vi "oa_Calculate Orbit Precession Direction.vi"(4 "revolutions":dbl format="%.2f", 5 "reset? (F)":bool, 6 "actual samples/rev":dbl format="%.2f", 7 "tach duty":i32=1, 8 "error in (no error)":errorcluster, 9 "max axis value":dbl format="%.2f", 10 "shaft rotating direction":u16, 11 "XY plot data in":cluster{dbl[], dbl[]}[](array[cluster]) {"?" format="%.2f"; "?" format="%.2f"}) -> (0 "error out":errorcluster, 1 "max value":dbl, 2 "orbit precession direction":u16(ring) items=["forward", "backward"], 3 "XY plot data out":cluster{dbl[], dbl[]}[](array[cluster]) {"?" format="%.2f"; "?" format="%.2f"})   [LabVIEW 2017]
uses:
  <vilib>/Analysis/1siggen.llb/Ramp Pattern by Samples.vi
  <vilib>/Analysis/NI_AALPro.lvlib
  <vilib>/Analysis/NI_AALBase.lvlib
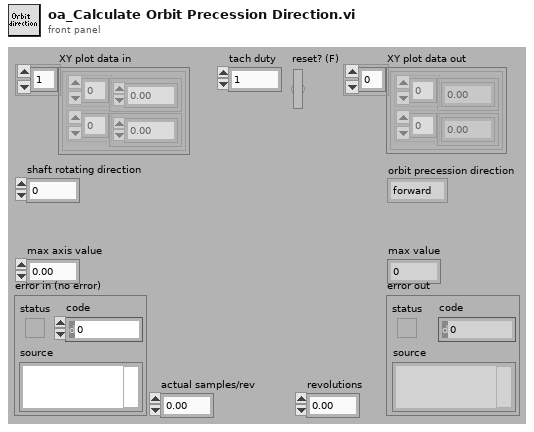
[diagram p1: front panel]
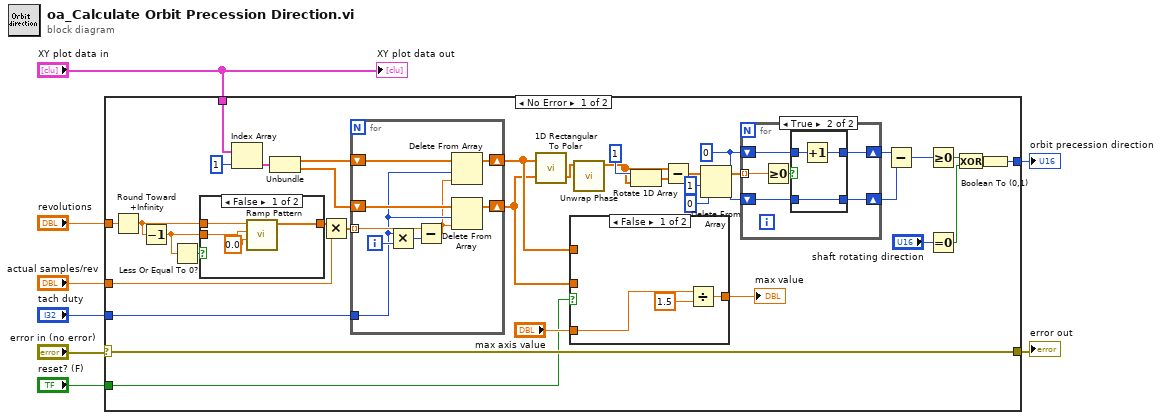
[diagram p0: block diagram]
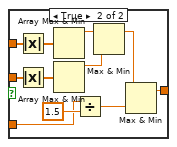
[diagram p2: hidden frame]
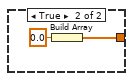
[diagram p3: hidden frame]
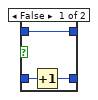
[diagram p4: hidden frame]
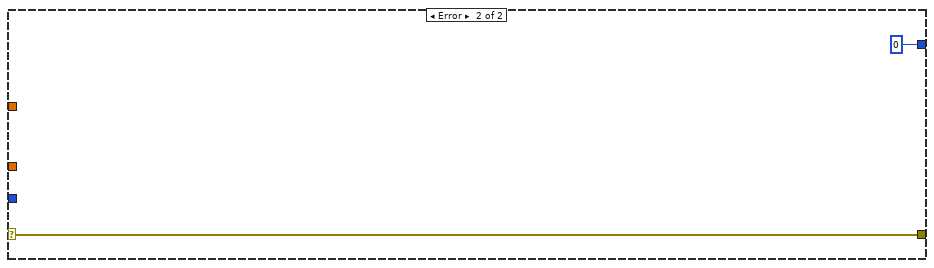
[diagram p5: hidden frame]
diagram:
  n1 = case shown="No Error" "error in (no error)" {
    selector: "error in (no error)" -> [w10 w87]
    tunnel: [w44 i16 0] -> w8
    tunnel: "XY plot data in" -> [w39 _]
    tunnel: "revolutions" -> [w24 _]
    tunnel: "tach duty" -> [w23 _]
    tunnel: "actual samples/rev" -> [w21 _]
    tunnel: [w10 w87] -> w2
    tunnel: "reset? (F)" -> [w9 _]
    frame No Error {
      w26 = 0
      n2 = Round Toward +Infinity(x=w24) -> (ceil(x): smallest int >= x=w13:dbl)
      n3 = Decrement(x=w13) -> (x-1=w11:dbl)
      n4 = Less Or Equal To 0?(x=w11) -> (x <= 0?=w12:bool)
      n5 = case shown="False" w12 {
        tunnel: w13 -> [w61 _]
        tunnel: w11 -> [w60 _]
        tunnel: [w59 w64] -> w20
        frame False {
          n6 = call-poly <vilib>:"Ramp Pattern.vi"("start"=0.0, "end"=w60, "samples"=w61) -> ("Ramp Pattern"=w59:dbl[])  [unwired: 7 in, 1 out]
        }
        frame True {
          n7 = Build Array(0.0 ("element")) -> (w64:dbl[])
        }
      }
      n8 = Index Array(array=w39, index=1) -> (element=w35:cluster{dbl[], dbl[]})
      n9 = Unbundle(w35) -> (w22:dbl[], w18:dbl[])
      n10 = Multiply(x=w20, y=w21) -> (x*y=w19:dbl[])
      n11 = for {
        tunnel: w23 -> [w66]
        shift-right: [w72] -> w17
        shift-left: w22 -> [w73]
        tunnel: w19 -> [w71] mode=indexing
        shift-right: [w67] -> w16
        shift-left: w18 -> [w68]
        i -> [w70]
        n12 = Multiply(x=w66, y=w70) -> (x*y=w69:i32)
        n13 = Subtract(x=w71, y=w69) -> (x-y=w65:dbl)
        n14 = Delete From Array(array=w73, length=w66, index=w65) -> (array with subset deleted=w72:dbl[])  [unwired: 1 out]
        n15 = Delete From Array(array=w68, length=w66, index=w65) -> (array with subset deleted=w67:dbl[])  [unwired: 1 out]
      }
      n16 = call <vilib>:"1D Rectangular To Polar.vi"("X"=w17, "Y"=w16) -> ("Phase"=w27:dbl[])  [unwired: 2 out]
      n17 = case shown="False" w9 {
        tunnel: "max axis value" -> [w47 w53]
        tunnel: [w45 w50] -> w36
        tunnel: w17 -> [_ w49]
        tunnel: w16 -> [_ w48]
        frame False {
          n18 = Divide(x=w47, y=1.5) -> (x/y=w45:dbl)
        }
        frame True {
          n19 = Absolute Value(x=w49) -> (abs(x)=w58:dbl[])
          n20 = Absolute Value(x=w48) -> (abs(x)=w57:dbl[])
          n21 = Array Max & Min(array=w58) -> (max value=w56:dbl)  [unwired: 3 out]
          n22 = Array Max & Min(array=w57) -> (max value=w55:dbl)  [unwired: 3 out]
          n23 = Divide(x=w53, y=1.5) -> (x/y=w52:dbl)
          n24 = Max & Min(x=w56, y=w55) -> (max(x,y)=w51:dbl)  [unwired: 1 out]
          n25 = Max & Min(x=w51, y=w52) -> (max(x,y)=w50:dbl)  [unwired: 1 out]
        }
      }
      "max value" <- w36
      n26 = call <vilib>:"Unwrap Phase.vi"("Phase"=w27) -> ("Unwrapped Phase"=w29:dbl[])  [unwired: 9 in, 1 out]
      n27 = Rotate 1D Array(1:w29, 2:1 ("n")) -> (0:w31:dbl[])
      n28 = Subtract(x=w29, y=w31) -> (x-y=w32:dbl[])
      n29 = Delete From Array(array=w32, length=1, index=0) -> (array with subset deleted=w28:dbl[])  [unwired: 1 out]
      n30 = for {
        tunnel: w28 -> [w79] mode=indexing
        shift-right: [w75] -> w15
        shift-left: w26 -> [w77]
        shift-right: [w74] -> w14
        shift-left: w26 -> [w76]
        n31 = Greater Or Equal To 0?(x=w79) -> (x >= 0?=w78:bool)
        n32 = case shown="True" w78 {
          tunnel: w77 -> [w82 w85]
          tunnel: w76 -> [w81 w83]
          tunnel: [w82 w84] -> w75
          tunnel: [w80 w83] -> w74
          frame False {
            n33 = Increment(x=w81) -> (x+1=w80:i32)
          }
          frame True {
            n34 = Increment(x=w85) -> (x+1=w84:i32)
          }
        }
      }
      n35 = Subtract(x=w15, y=w14) -> (x-y=w38:i32)
      n36 = Greater Or Equal To 0?(x=w38) -> (x >= 0?=w41:bool)
      n37 = Equal To 0?(x="shaft rotating direction") -> (x = 0?=w42:bool)
      n38 = Exclusive Or(1:w42, 2:w41) -> (0:w43:bool)
      n39 = Boolean To (0,1)(Boolean=w43) -> (0, 1=w44:i16)
    }
    frame Error {
    }
  }
  "orbit precession direction" <- w8
  "error out" <- w2
  "XY plot data out" <- "XY plot data in"
